vi "Read Finance Data.vi"() -> (0 "Result Array":string[][](array[string]), 3 "Line Size":dbl[](array[numeric]) format="%#_1g")   [LabVIEW 2023]
uses:
  <vilib>/Utility/file.llb/Read Delimited Spreadsheet (string).vi
panel:
  out "Array 2":string[](array[string])
  out "substring":string
  out "number":i32
  out "String 2":string
  out "spreadsheet string":string
  out "Array":string[][](array[string])
  out "all rows":string[][](array[string])
  out "match + rest of string":string
  out "substring before match":string
  out "String":string
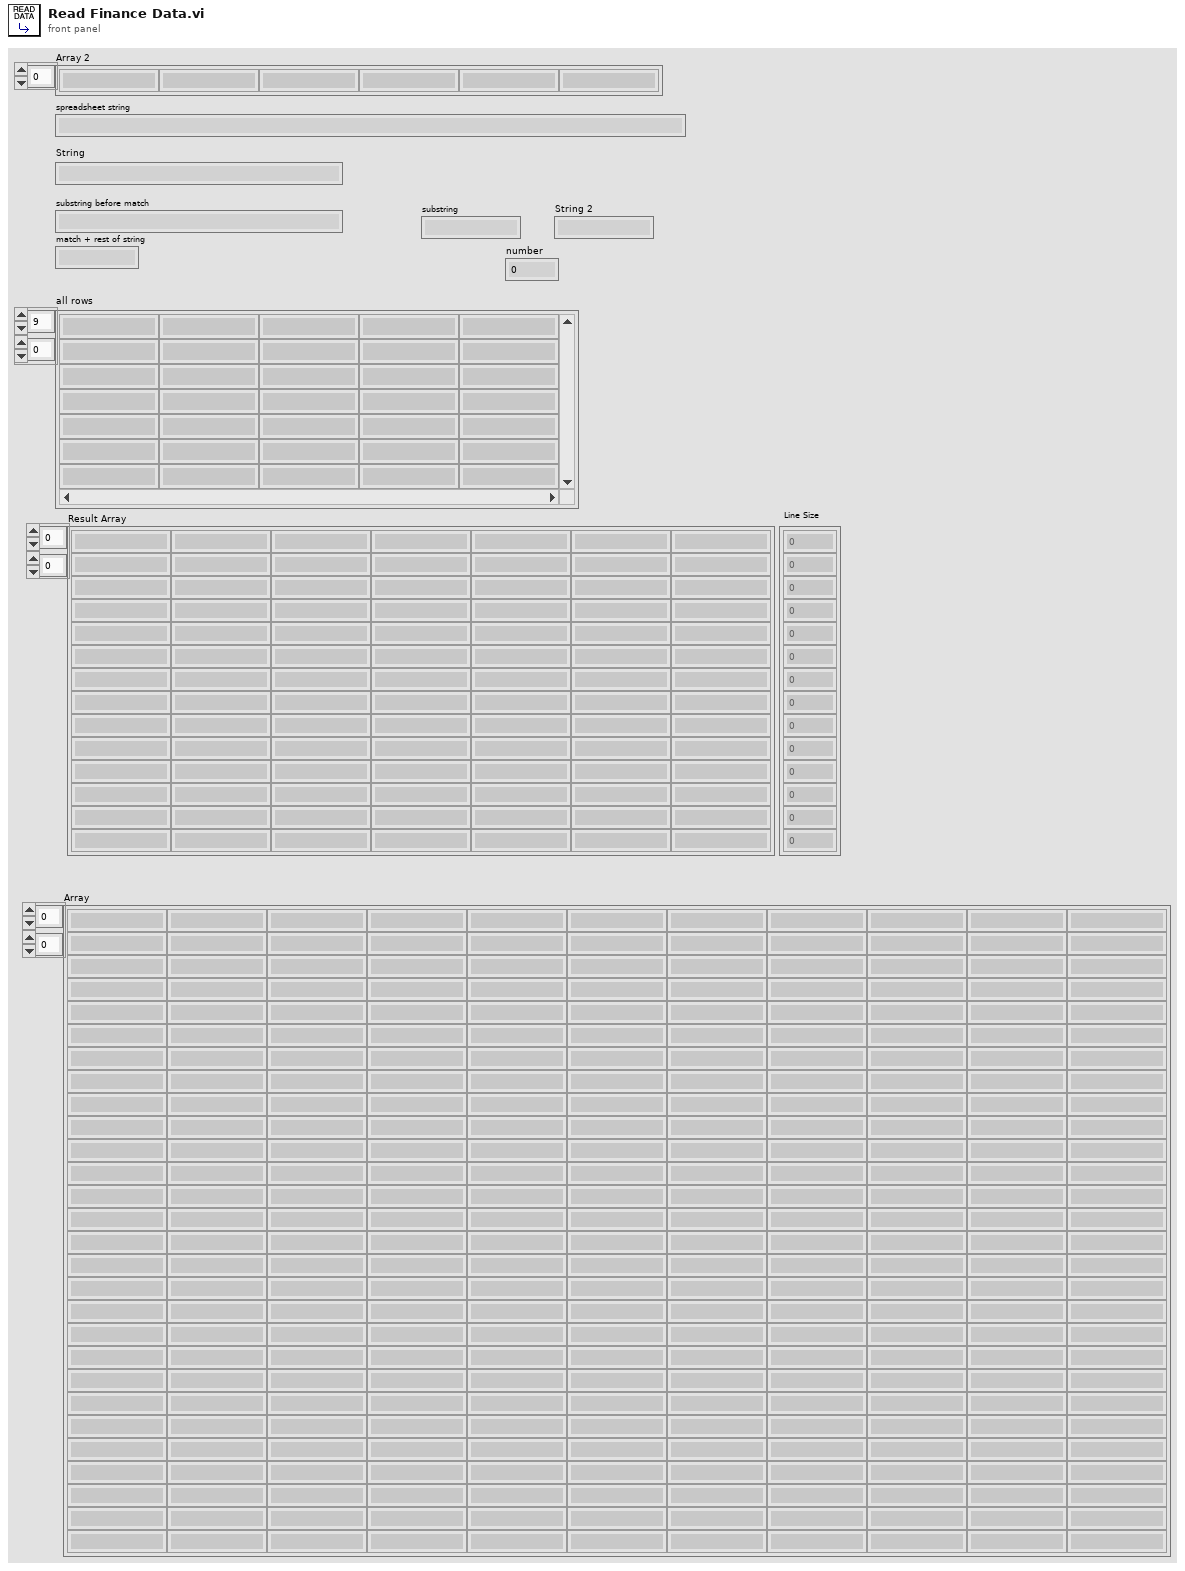
[diagram p1: front panel]
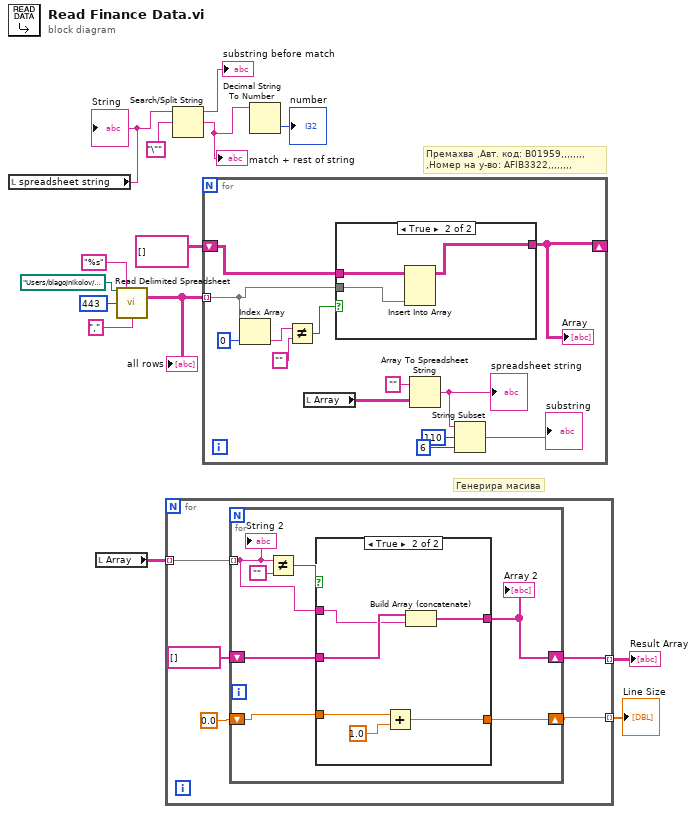
[diagram p0: block diagram]
diagram:
  # "Генерира масива"
  # "Премахва ,Авт. код: B01959,,,,,,,,\n,Номер на у-во: AFIB3322,,,,,,,,"
  n1 = local read "spreadsheet string"() -> (w6:string)
  "String" <- w6
  n2 = local read "Array"() -> (w5:string[][])
  n3 = call-poly <vilib>:"Read Delimited Spreadsheet.vi"("file path (dialog if empty)"=path "/Users/blagojnikolov/Documents/VSCode/report.csv" ("file (use dialog)"), "format (%s)"="%s" ("format (%.3f)"), "start of read offset (chars.:0)"=443, "delimiter (\\t)"="," ("delimiter (\\t)")) -> ("all rows"=w9:string[][])  [unwired: 6 in, 5 out]
  "all rows" <- w9
  n4 = for {
    tunnel: w5 -> [w19] mode=indexing
    tunnel: [w17] -> w2 mode=indexing
    tunnel: [w15] -> w1 mode=indexing
    n5 = for {
      tunnel: w19 -> [w23] mode=indexing
      shift-right: [w22] -> w17
      shift-left: string[] [] -> [w24]
      shift-right: [w21] -> w15
      shift-left: 0.0 -> [w20]
      n6 = Not Equal?(x=w23, y="") -> (x != y?=w26:bool)
      n7 = case shown="True" w26 {
        tunnel: [w28 w34] -> w22
        tunnel: w24 -> [w28 w33]
        tunnel: w23 -> [_ w32]
        tunnel: [w27 w30] -> w21
        tunnel: w20 -> [w27 w29]
        frame False {
        }
        frame True {
          n8 = Add(x=w29, y=1.0) -> (x+y=w30:dbl)
          n9 = Build Array (concatenate)(w33, w32) -> (w34:string[])
        }
      }
      "Array 2" <- w22
      "String 2" <- w23
    }
  }
  "Result Array" <- w2
  "Line Size" <- w1
  n10 = Search/Split String(string=w6, search string/char (-)="\"") -> (substring before match=→"substring before match":string, match + rest of string=w4:string)  [unwired: 1 in, 1 out]
  "match + rest of string" <- w4
  n11 = for {
    tunnel: w9 -> [w41] mode=indexing
    shift-right: [w42] -> _
    shift-left: string[][] [] -> [w44]
    n12 = Index Array(array=w41, index=0) -> (element=w43:string)
    n13 = Not Equal?(x=w43, y="") -> (x != y?=w45:bool)
    n14 = local read "Array"() -> (w39:string[][])
    n15 = case shown="True" w45 {
      tunnel: [w48 w51] -> w42
      tunnel: w44 -> [w48 w50]
      tunnel: w41 -> [_ w49]
      frame False {
      }
      frame True {
        n16 = Insert Into Array(array=w50, new element=w49) -> (w51:string[][])  [unwired: 2 in]
      }
    }
    "Array" <- w42
    n17 = Array To Spreadsheet String(array=w39, 3:"" ("format string")) -> (spreadsheet string=w38:string)  [unwired: 1 in]
    "spreadsheet string" <- w38
    n18 = String Subset(string=w38, offset (0)=110, length (rest)=6 ("length (rest)")) -> (substring=→"substring":string)
  }
  n19 = Decimal String To Number(string=w4) -> (number=→"number":i32)  [unwired: 2 in, 1 out]
